vi "Sequence-Start.vi"(8 "error in (no error)":errorcluster, 10 "SeqOptions":T1) -> (0 "error out":errorcluster)   [LabVIEW 2016]
uses:
  Sequence.UserData.ctl
  Sequence.MainMode.ctl
  Gui/MainGui.TestOptions.ctl
  Sequence.Action.ctl
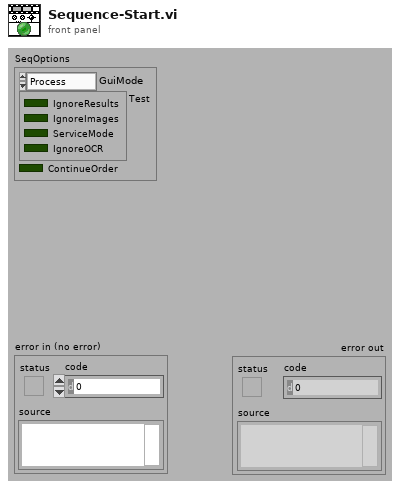
[diagram p1: front panel]
types:
  T1 = typedef "Sequence.UserData.ctl" = cluster{"GuiMode":T2, "Test":T3, "ContinueOrder":bool}
  T2 = typedef "Sequence.MainMode.ctl" = enum16{"Process", "Base", "Order", "Manual", "Logs", "Results", "Stats", "DMC Config"}
  T3 = typedef "MainGui.TestOptions.ctl" = cluster{"IgnoreResults":bool, "IgnoreImages":bool, "ServiceMode":bool, "IgnoreOCR":bool}
  T4 = typedef "Sequence.Action.ctl" = enum32{"idle", "constructor", "destructor", "--- Sequence ---", "Abort", "Init", "Select", "Start", "Work.Run", "Work.AirON", "Work.LaserON", "Work.Done", "Process.Run", "Process.Engine", "Process.Pause", "Process.DoorLock", "Process.Wait4Container", "Process.Wait1", "Process.Wait2", "Process.Continue", "Process.Done", "Home.Run", "Home.AirON", "Home.TablePos", "Home.MoveServo", "Home.LaserOFF", "Home.AirOFF", "Home.Done", "User.Action", "User.Data", "Status.Clear"}
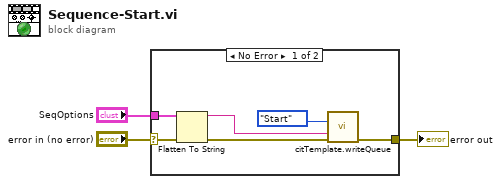
[diagram p0: block diagram]
diagram:
  n1 = case shown="No Error" "error in (no error)" {
    selector: "error in (no error)" -> [w7 w10]
    tunnel: [w9 w10] -> w2
    tunnel: "SeqOptions" -> [w4 _]
    frame No Error {
      n2 = Flatten To String(anything=w4, error in (no error)=w7) -> (data string=w5:string, error out=w6:errorcluster)  [unwired: 2 in, 1 out]
      n3 = call "citTemplate.writeQueue.vi"("event in (if not connected:all statemachine with data event)"=Sequence.Action."Start" ("Action"), "data in"=w5, "error in (no error)"=w6) -> ("error out"=w9:errorcluster)  [unwired: 12 in]
    }
    frame Error {
    }
  }
  "error out" <- w2
